vi "skip_status.vi"() -> ()   [LabVIEW 2020]
panel:
  in  "skip_status":bool
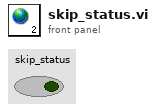
[diagram p1: front panel]
diagram:
